vi "Read_File_Simple.vi"(0 "Filename":path, 1 "number of characters (all:-1)":i32=-1, 3 "pos offset (bytes:0)":i32) -> (5 "error out":errorcluster, 6 "Error?":bool, 7 "Filename Out":path, 8 "string":string, 9 "EOF?":bool, 10 "mark after read (chars.)":i32)   [LabVIEW 2010]
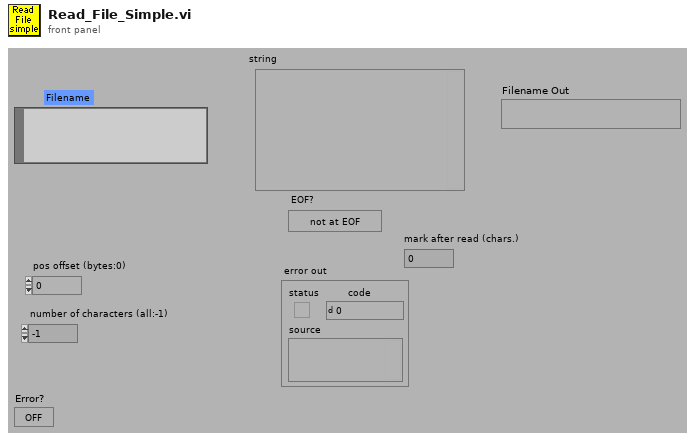
[diagram p1: front panel]
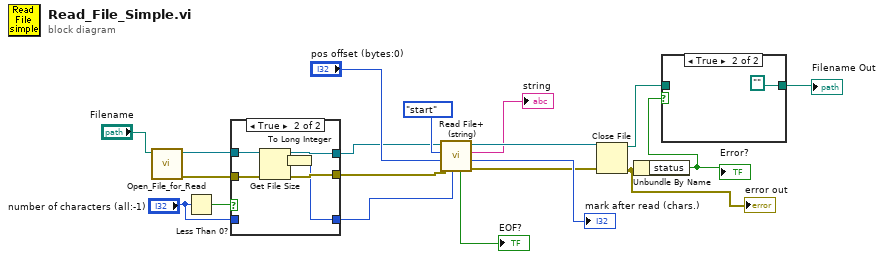
[diagram p0: block diagram]
diagram:
  n1 = call "Open_File_for_Read.vi"("file path"="Filename") -> ("error out"=w1:errorcluster, "refnum"=w2:refnum<file>)  [unwired: 9 out]
  n2 = Less Than 0?(x="number of characters (all:-1)") -> (x < 0?=w12:bool)
  n3 = case shown="True" w12 {
    tunnel: w2 -> [w22 w28]
    tunnel: w1 -> [w21 w27]
    tunnel: [w21 w26] -> w11
    tunnel: [w22 w25] -> w10
    tunnel: [w20 w24] -> w9
    tunnel: "number of characters (all:-1)" -> [w20 _]
    frame False {
    }
    frame True {
      n4 = Get File Size(file=w28, error in=w27) -> (refnum out=w25:refnum<file>, size (in bytes)=w23:i64, 0:w26:errorcluster)
      n5 = To Long Integer(number=w23) -> (32bit integer=w24:i32)
    }
  }
  n6 = call <vilib>:"Read File+ (string).vi"("count"=w9, "error in (no error)"=w11, "pos offset (bytes:0)"="pos offset (bytes:0)", "pos mode (rel. to current:2)"=enum16{"start", "end", "current"}."start", "refnum"=w10) -> ("error out"=w15:errorcluster, "mark after read (bytes)"=→"mark after read (chars.)":i32, "string"=→"string":string, "dup refnum"=w16:refnum<file>, "EOF?"=→"EOF?":bool)  [unwired: 2 out]
  n7 = Close File(refnum=w16, error in=w15) -> (path=w4:path, error out=w7:errorcluster)
  "error out" <- w7
  n8 = Unbundle By Name(w7) -> ("status"=w6:bool)
  "Error?" <- w6
  n9 = case shown="True" w6 {
    tunnel: [w29 path ""] -> w5
    tunnel: w4 -> [w29 _]
    frame False {
    }
    frame True {
    }
  }
  "Filename Out" <- w5
